vi "dosimat_load_command.vi"(2 "error in":errorcluster, 3 "Method":string="Fill", 4 "Dosimat Port In":refnum<visa-resource-name>="COM1") -> (0 "error out":errorcluster, 1 "Dosimat Port Out":refnum<visa-resource-name>="COM1")   [LabVIEW 2010]
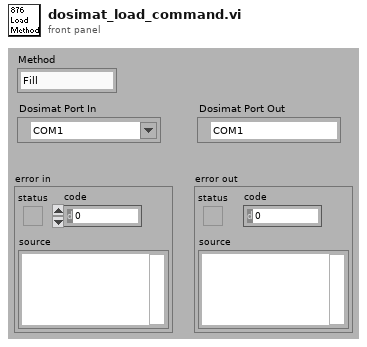
[diagram p1: front panel]
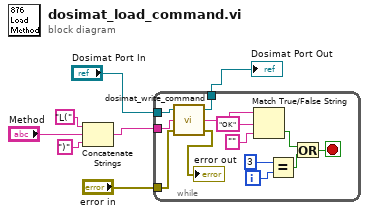
[diagram p0: block diagram]
diagram:
  n1 = Concatenate Strings("L(" ("string"), "Method", ")" ("string")) -> (w6:string)
  n2 = while {
    tunnel: "Dosimat Port In" -> [w20]
    tunnel: w6 -> [w10]
    tunnel: "error in" -> [w9]
    tunnel: [w8] -> w1
    i -> [w18]
    stop <- w16 stop-if-true
    n3 = call "dosimat_write_command.vi"("error in"=w9, "write buffer"=w10, "Dosimat Port In"=w20) -> ("error out"=→"error out":errorcluster, "read buffer"=w19:string, "Dosimat Port Out"=w8:refnum<visa-resource-name>)
    n4 = Match True/False String(2:"" ("false string"), 3:"OK" ("true string"), 4:w19) -> (0:w15:bool)  [unwired: 1 out]
    n5 = Equal?(x=3, y=w18) -> (x = y?=w14:bool)
    n6 = Or(x=w15, y=w14) -> (x .or. y?=w16:bool)
  }
  "Dosimat Port Out" <- w1
